vi "testUnsupportedType.vi"() -> ()   [LabVIEW 2019, in "TestSuiteTest.lvlib" / "Create.lvlib"]
uses:
  Create.lvlib
  TestSuite/TestSuite.lvclass
  Assertion/Assertion.lvlib
panel:
  out "error out":errorcluster
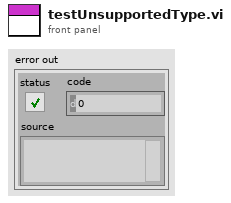
[diagram p1: front panel]
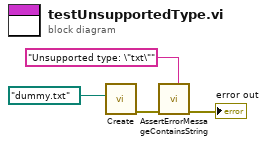
[diagram p0: block diagram]
diagram:
  n1 = call "Create.vi"("Path"=path "dummy.txt") -> ("error out"=w4:errorcluster)  [unwired: 9 in, 1 out]
  n2 = call "AssertErrorMessageContainsString.vi"("Expected"="Unsupported type: \"txt\"", "error in (no error)"=w4) -> ("error out"=→"error out":errorcluster)  [unwired: 9 in]
